vi "MH_ReadFiFo.vi"(8 "error in (no error)":errorcluster, 11 "devidx":i32) -> (0 "error out":errorcluster, 1 "nactual":i32, 2 "buffer":u32[](array[numeric]), 3 "return type":i32)   [LabVIEW 2019]
uses:
  MH_DllPath_global.vi
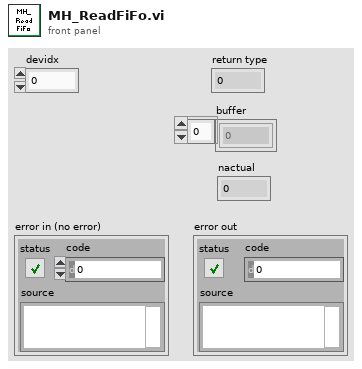
[diagram p1: front panel]
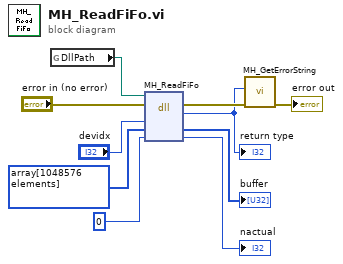
[diagram p0: block diagram]
diagram:
  n1 = global read "MH_DllPath_global.vi" "DllPath"() -> (w9:path)
  n2 = dll-call lib="MHLib64.dll" fn="MH_ReadFiFo"(path in=w9, error in="error in (no error)", "devidx"="devidx", "buffer"=u32[] array[1048576 elements], "nactual"=0) -> (error out=w7:errorcluster, "return type"=w6:i32, "buffer"=→"buffer":u32[], "nactual"=→"nactual":i32)  [unwired: 2 in, 1 out]
  "return type" <- w6
  n3 = call "MH_GetErrorString.vi"("error in (no error)"=w7, "code"=w6) -> ("error out"=→"error out":errorcluster)  [unwired: 7 in, 2 out]
